vi "TagDB-Set Lock.vi"(8 "error in (no error)":errorcluster, 10 "Lock?(T)":bool=TRUE, 11 "TagDB":T1) -> (0 "error out":errorcluster, 3 "TagDB(dup)":T1)   [LabVIEW 2017, in "TagDB.lvlib"]
uses:
  TagDB.lvlib
  Typedef/TagDB.ctl
  _Support/Error/_Build Error Cluster.vi
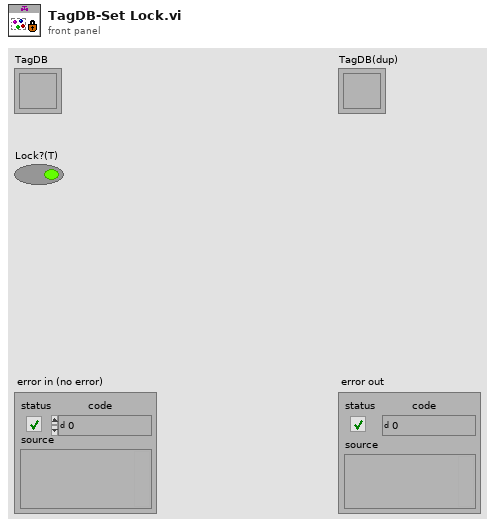
[diagram p1: front panel]
types:
  T1 = typedef "TagDB.lvlib/TagDB.ctl" = refnum<k1>
  T2 = typedef "TagContainer(DEV).lvlib/tagcontainer-data.ctl" = cluster{"tag-map":variant, "timestamp-map":variant, "namecacher-map":variant, "DataTypeCacher-map":variant, "Tag Adding Lock?":bool, "Global Change Timestamp":timestamp, "Item Change Timestamp":timestamp, "name":string}
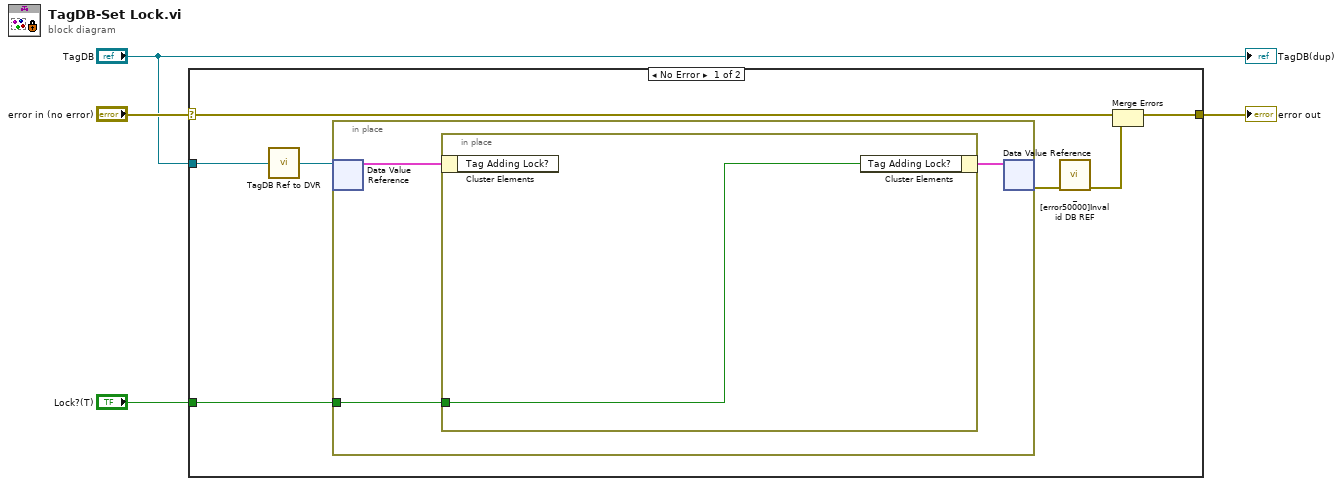
[diagram p0: block diagram]
diagram:
  n1 = case shown="No Error" "error in (no error)" {
    selector: "error in (no error)" -> [w10 w16]
    tunnel: [w11 w16] -> w3
    tunnel: "TagDB" -> [w8 _]
    tunnel: "Lock?(T)" -> [w6 _]
    frame No Error {
      n2 = call "TagDB Ref to DVR.vi"("TagDB"=w8) -> ("DVR"=w7:refnum<data-value>)  [unwired: 4 in]
      n3 = in-place "In Place Element Structure" {
        in-place-border: w6 -> [w14]
        n4 = in-place-dvr #1(w7) -> (w13:T2)  [unwired: 1 out]
        n5 = in-place {
          in-place-border: w14 -> [w15]
          n6 = in-place-cluster #2(w13) -> ()  [unwired: 1 out]
          n7 = in-place-cluster #2("Tag Adding Lock?"=w15) -> (w12:T2)
        }
        n8 = in-place-dvr #1(w12) -> (w9:errorcluster)  [unwired: 1 out]
      }
      n9 = call "_[error50000]Invalid DB REF.vi"("error in (no error)"=w9) -> ("error out"=w5:errorcluster)  [unwired: 10 in]
      n10 = Merge Errors(w10, w5) -> (w11:errorcluster)
    }
    frame Error {
    }
  }
  "error out" <- w3
  "TagDB(dup)" <- "TagDB"
